vi "Actor Core.vi"(8 "error in":errorcluster, 11 "Cam_SLM_Controller in":refnum<class "Cam_SLM_Controller.lvclass">) -> (0 "error out":errorcluster, 3 "Actor out":refnum<class "Actor.lvclass">)   [LabVIEW 2023, in "Cam_SLM_controller.lvlib" / "Cam_SLM_Controller.lvclass"]
doc: "(<B>Filename</B>: Actor Framework.lvlib:Actor.lvclass:Actor Core.vi)\n\nReceives messages to the actor, reacts to them, and initiates any error handling that may shut the actor down.\n\nDescendant classes may override this VI to append parallel tasks for the actor to complete while it handles messages. Overrides use the Call Parent Class Method node."
uses:
  Cam_SLM_Controller.lvclass
  <vilib>/ActorFramework/Actor/Actor.lvclass
  UIs/SLM_Controller/SLM_Controller/SLM_Controller/SLM_Controller.lvclass
  UIs/Camera_Controller/Camera_Controller/Camera_Controller.lvclass
  Cam_SLM_Controller.lvclass/Cam_SLM_Controller.ctl
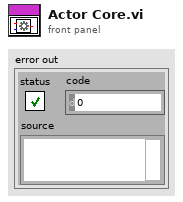
[diagram p1: front panel]
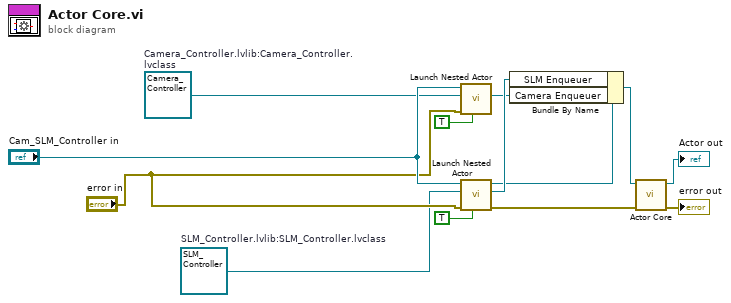
[diagram p0: block diagram]
diagram:
  w4 = refnum<class "Camera_Controller.lvclass"> refnum  # Camera_Controller.lvlib:Camera_Controller.lvclass
  w7 = refnum<class "SLM_Controller.lvclass"> refnum  # SLM_Controller.lvlib:SLM_Controller.lvclass
  n1 = call <vilib>:"Launch Nested Actor.vi"("Open Actor Core front panel? (F)"=TRUE, "error in (no error)"="error in", "Nested Actor"=w4, "Caller Actor in"="Cam_SLM_Controller in") -> ("Nested Actor's Enqueuer"=w3:refnum<class "Message Enqueuer.lvclass">)  [unwired: 5 in, 2 out]
  n2 = call <vilib>:"Launch Nested Actor.vi"("Open Actor Core front panel? (F)"=TRUE, "error in (no error)"="error in", "Nested Actor"=w7, "Caller Actor in"="Cam_SLM_Controller in") -> ("error out"=w11:errorcluster, "Nested Actor's Enqueuer"=w6:refnum<class "Message Enqueuer.lvclass">, "Caller Actor out"=w5:refnum<class "Cam_SLM_Controller.lvclass">)  [unwired: 5 in]
  n3 = Bundle By Name(cluster=w5, "SLM Enqueuer"=w6, "Camera Enqueuer"=w3) -> (w10:refnum<class "Cam_SLM_Controller.lvclass">)
  n4 = call-parent "Actor Core.vi"("error in"=w11, "Actor in"=w10) -> ("error out"=→"error out":errorcluster, "Actor out"=→"Actor out":refnum<class "Actor.lvclass">)  [unwired: 8 in]
